vi "Set Current.vi"(8 "error in (no error)":errorcluster, 9 "Shot":i32, 10 "Tree name":string, 11 "Tree in":refnum<class "Tree.lvclass">) -> (0 "error out":errorcluster, 3 "Tree out":refnum<class "Tree.lvclass">)   [LabVIEW 2013, in "MDSplus.lvlib" / "Tree.lvclass"]
doc: "Set the current tree and shot."
uses:
  <vilib>/MDSplus/Classes/Tree_Class/Tree.lvclass
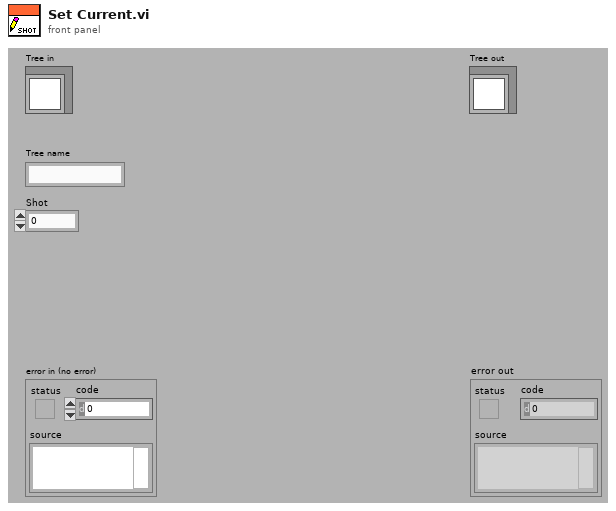
[diagram p1: front panel]
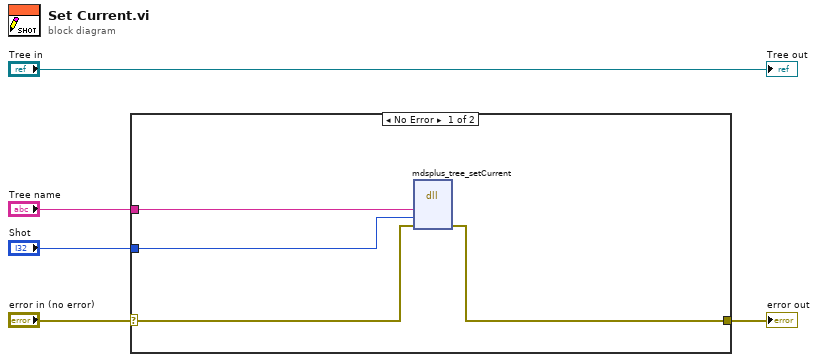
[diagram p0: block diagram]
diagram:
  n1 = case shown="No Error" "error in (no error)" {
    selector: "error in (no error)" -> [w7 w10]
    tunnel: [w6 w10] -> w4
    tunnel: "Tree name" -> [w9 _]
    tunnel: "Shot" -> [w8 _]
    frame No Error {
      n2 = dll-call lib="MDSobjectsLVShr" fn="mdsplus_tree_setCurrent"("treeNameIn"=w9, "shotIn"=w8, "error"=w7) -> ("error"=w6:errorcluster)  [unwired: 6 in, 2 out]
    }
    frame Error {
    }
  }
  "error out" <- w4
  "Tree out" <- "Tree in"
